vi "Get the class reference.vi"() -> (0 "ChildClass.lvclass":refnum<class "ChildClass.lvclass">)   [LabVIEW 2022 SP3, in "ChildClass.lvclass"]
uses:
  ChildClass.lvclass
  ChildClass.lvclass/ChildClass.ctl
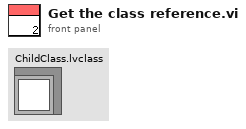
[diagram p1: front panel]
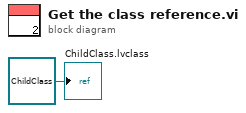
[diagram p0: block diagram]
diagram:
  "ChildClass.lvclass" <- refnum<class "ChildClass.lvclass"> refnum ("ChildClass.lvclass")
